vi "GetLGRDigitMap.vi"(8 "error in (no error)":errorcluster, 11 "EAN-13 in":refnum<class "EAN-13.lvclass">) -> (0 "error out":errorcluster, 2 "LGR digit map":u8[][](array[numeric]), 3 "EAN-13 out":refnum<class "EAN-13.lvclass">)   [LabVIEW 2013, in "BarCodes.lvlib" / "EAN-13.lvclass"]
uses:
  EAN-13.lvclass
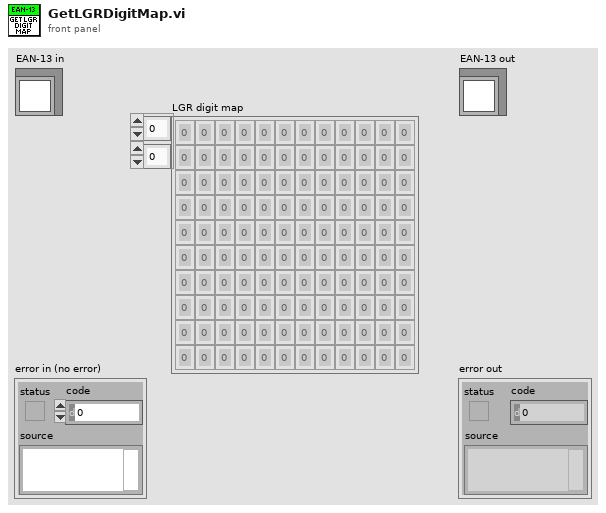
[diagram p1: front panel]
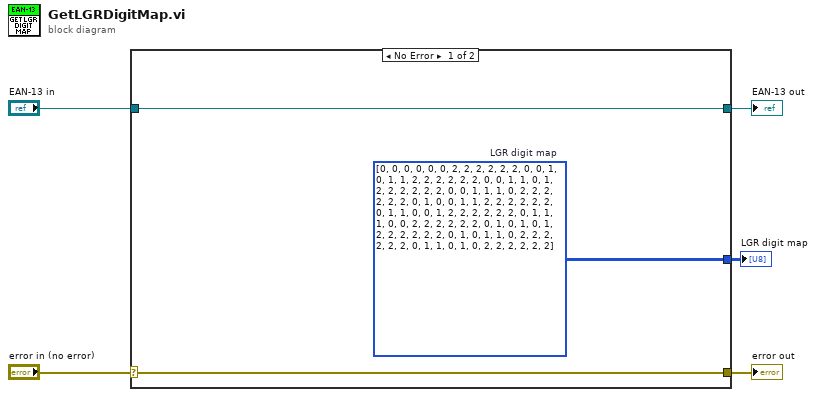
[diagram p0: block diagram]
diagram:
  n1 = case shown="No Error" "error in (no error)" {
    selector: "error in (no error)" -> [w7 w10]
    tunnel: [w7 w10] -> w4
    tunnel: [w8 w9] -> w2
    tunnel: "EAN-13 in" -> [w8 w9]
    tunnel: [w6 _] -> w1
    frame No Error {
      w6 = u8[][] [[0, 0, 0, 0, 0, 0, 2, 2, 2, 2, 2, 2], [0, 0, 1, 0, 1, 1, 2, 2, 2, 2, 2, 2], [0, 0, 1, 1, 0, 1, 2, 2, 2, 2, 2, 2], [0, 0, 1, 1, 1, 0, 2, 2, 2, 2, 2, 2], [0, 1, 0, 0, 1, 1, 2, 2, 2, 2, 2, 2], [0, 1, 1, 0, 0, 1, 2, 2, 2, 2, 2, 2], [0, 1, 1, 1, 0, 0, 2, 2, 2, 2, 2, 2], [0, 1, 0, 1, 0, 1, 2, 2, 2, 2, 2, 2], [0, 1, 0, 1, 1, 0, 2, 2, 2, 2, 2, 2], [0, 1, 1, 0, 1, 0, 2, 2, 2, 2, 2, 2]]  # LGR digit map
    }
    frame Error {
    }
  }
  "error out" <- w4
  "EAN-13 out" <- w2
  "LGR digit map" <- w1
